vi "Last_check.vi"(3 "error in":errorcluster, 4 "Step Number in":i32, 5 "Data in":T1) -> (0 "error out":errorcluster, 1 "Step Number out":i32, 2 "Data out":T1)   [LabVIEW 2017, in "Steps.lvlib"]
uses:
  Steps.lvlib
  Type_Defs/Data.ctl
  Type_Defs/Diagnostics.ctl
  Type_Defs/Systems.ctl
panel:
  in  "Step Back":bool
  in  "Continue":bool
  out "All Systems Ready?":bool=TRUE
  # "Options"
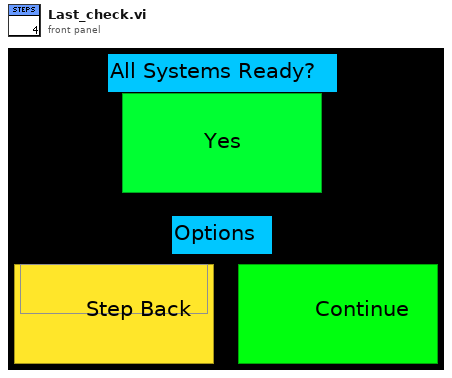
[diagram p1: front panel]
types:
  T1 = typedef "Data.ctl" = cluster{"User Name":string, "Experiment Number":i32, "Start Time":timestamp, "Data":dbl[], "Step Number":i32, "Step Instructions":string, "Diagnostics":T2, "Experiment Purpose":string, "Experiment State":enum16{"Off", "Setting Up", "Ready", "In Progress", "Shutting Down"}, "Systems":T3, "Vacuum Pressure":dbl, "Fieldpoints":cluster{"System Boolean Fieldpoints":cluster{"Compressed Air":refnum<k21>, "T-20kV Power Switch":refnum<k21>, "T-Rectifier":refnum<k21>, "Engage Interlock":refnum<k21>, "Ventilator":refnum<k21>, "Magnetron":refnum<k21>, "H-20kV Power Switch":refnum<k21>, "H-Rectifier":refnum<k21>, "Main Water Pump":refnum<k21>, "WEGA Water Pump":refnum<k21>, "Gas Inlet Valves":refnum<k21>}, "Step Fieldpoints":cluster{"Exhaust Ventillator":refnum<k21>, "Compressed Air":refnum<k21>, "Water Pressure":refnum<k21>, "Interlock":refnum<k21>, "Toroidal Power Supply 1":refnum<k21>, "Toroidal Power Supply 2":refnum<k21>, "Toroidal Rectifier":refnum<k21>, "Helical Power Supply":refnum<k21>, "Helical Rectifier":refnum<k21>, "6kW Magnetron Standby":refnum<k21>, "20kW Magnetron Standby":refnum<k21>}}, "Pressure History":cluster{"Seconds into Experiment":i32[], "Pressure Data":dbl[]}, "Time Computer Control":dbl[], "Toroidal Voltage Computer Control":dbl[], "Helical Voltage Computer Control":dbl[], "Toroidal Current":dbl[], "Toroidal Voltage":dbl[], "Toroidal Current Set Point":dbl[], "Helical Current Set Point":dbl[], "Helical Voltage":dbl[], "Helical Current":dbl[]}
  T2 = typedef "Diagnostics.ctl" = cluster{"Langmuir Probe":bool, "Rogowski 1":bool, "Rogowski 2":bool, "Rogowski 3":bool, "B-dot 1":bool, "B-dot 2":bool}
  T3 = typedef "Systems.ctl" = cluster{"Compressed Air":bool, "T-20kV Power Switch":bool, "T-Rectifier":bool, "Engage Interlock":bool, "Ventilator":bool, "Magnetron":bool, "H-20kV Power Switch":bool, "H-Rectifier":bool, "Main Water Pump":bool, "WEGA Water Pump":bool, "Gas Inlet Valves":bool}
  T4 = enum16{"Off", "Setting Up", "Ready", "In Progress", "Shutting Down"}
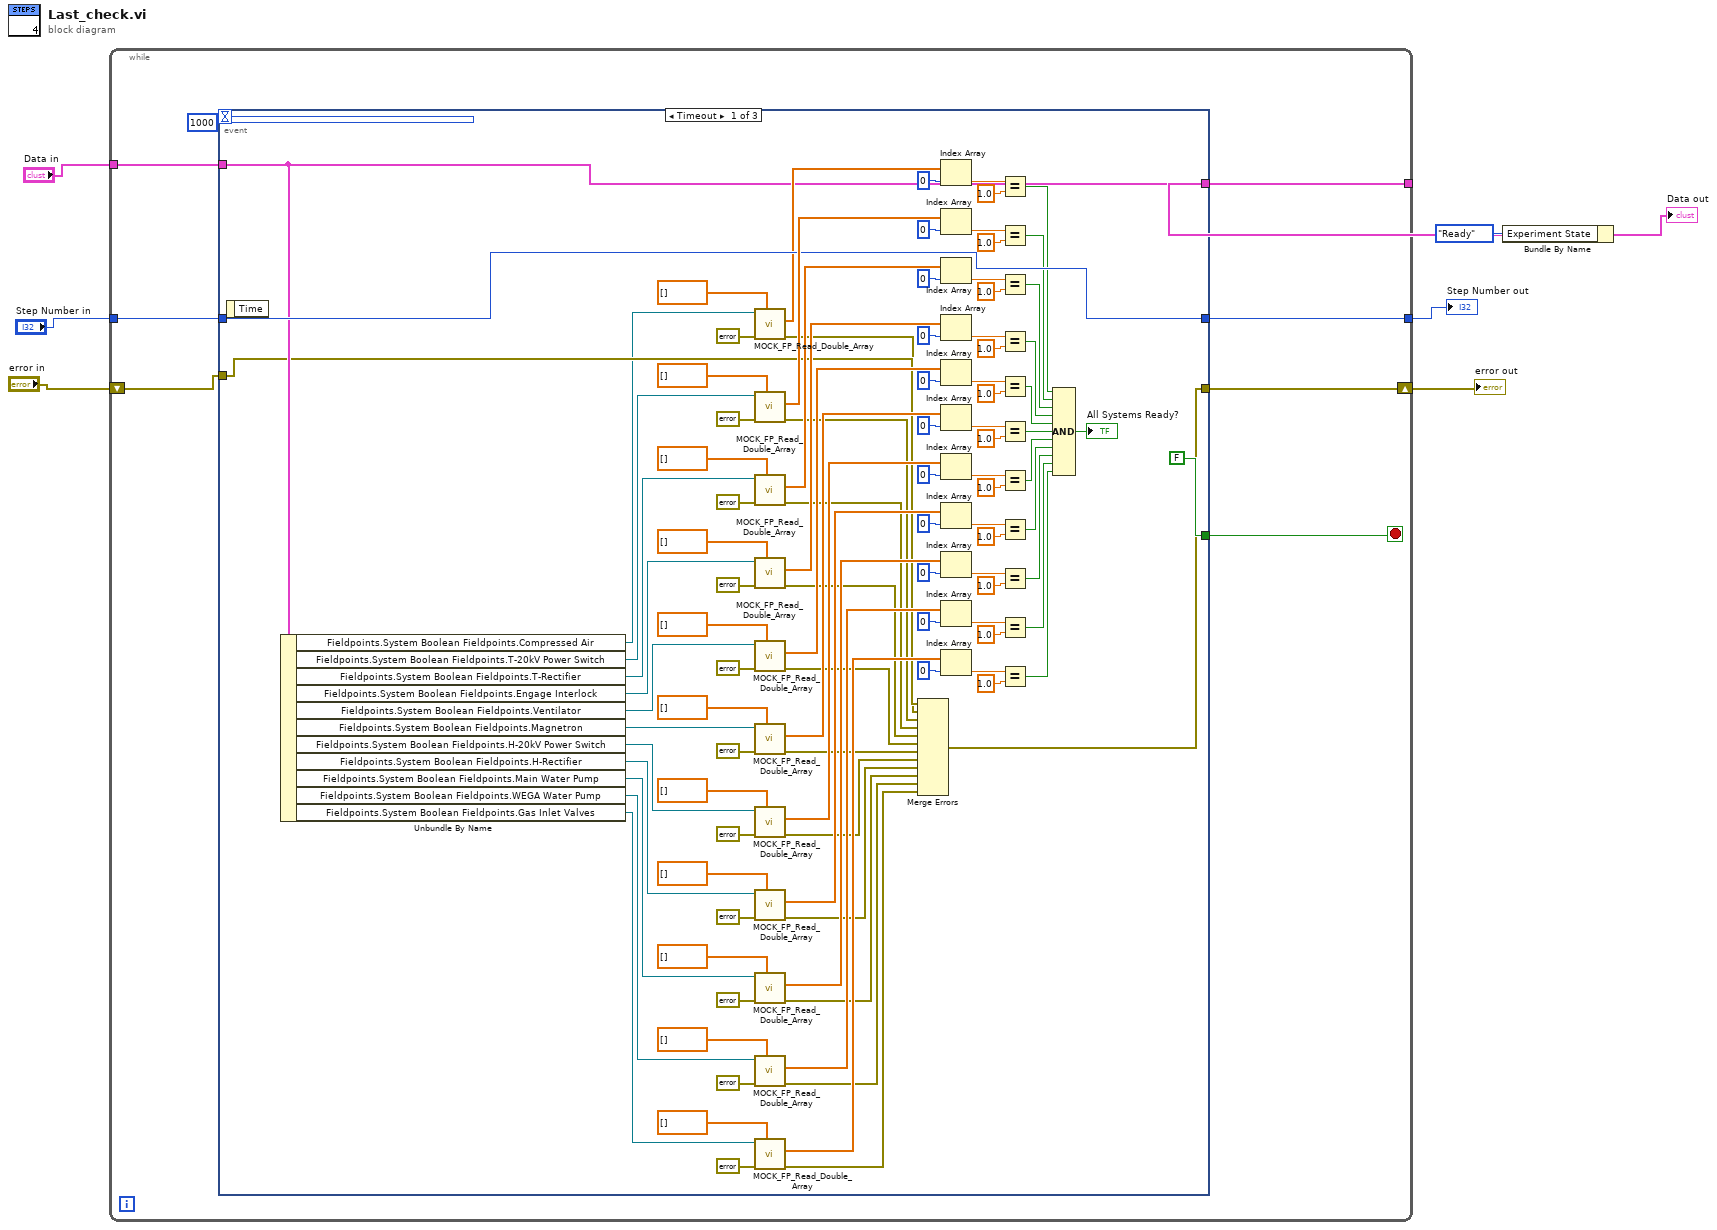
[diagram p0: block diagram]
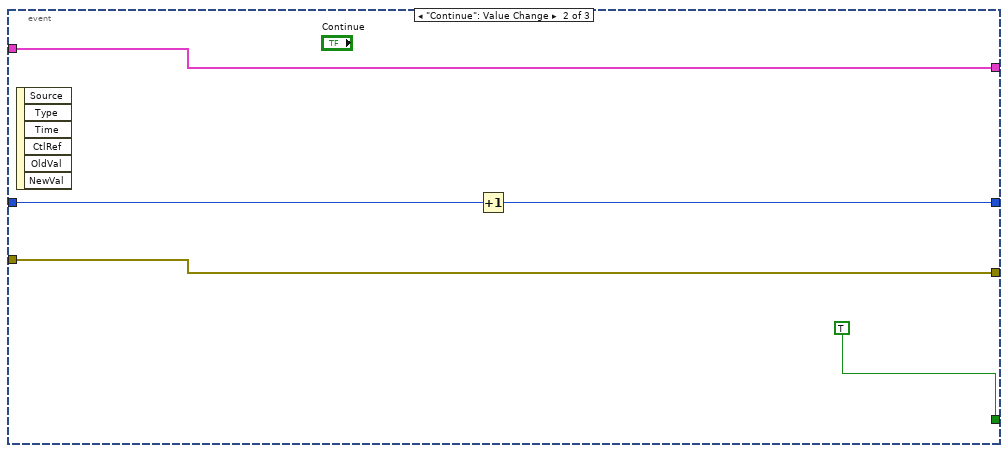
[diagram p2: hidden frame]
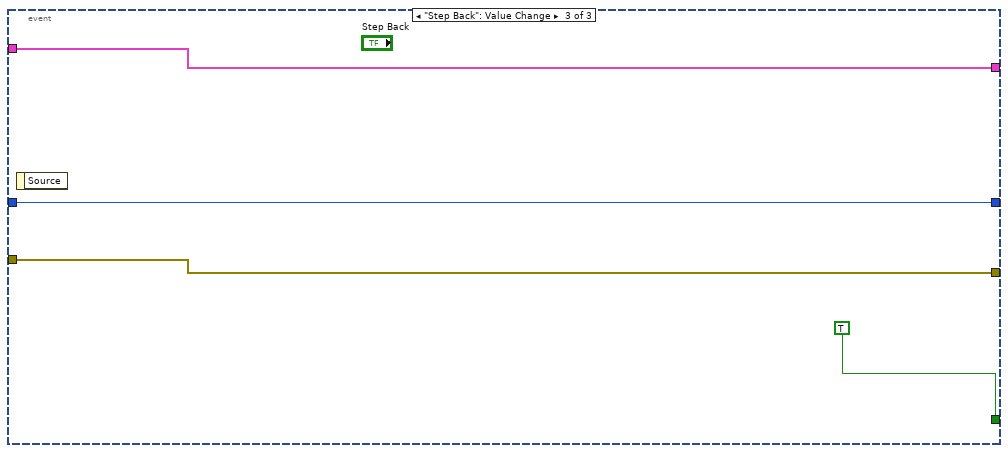
[diagram p3: hidden frame]
diagram:
  n1 = while {
    tunnel: [w12] -> w3
    tunnel: "Data in" -> [w11]
    tunnel: [w10] -> w6
    tunnel: "Step Number in" -> [w9]
    shift-right: [w14] -> w7
    shift-left: "error in" -> [w15]
    stop <- w13 stop-if-true
    n2 = event shown="[0] Timeout" {
      selector: _ -> [_ _ _]
      dyn-events: _ -> [_ _ _]
      timeout: 1000 -> [_ _ _]
      tunnel: w15 -> [w63 w125 w129]
      tunnel: [w62 w125 w129] -> w14
      tunnel: [FALSE TRUE TRUE] -> w13
      tunnel: [w64 w126 w130] -> w12
      tunnel: w11 -> [w64 w126 w130]
      tunnel: [w117 w123 w128] -> w10
      tunnel: w9 -> [w117 w124 w128]
      event Timeout {
        n3 = event-data() -> ()  [unwired: 1 in, 1 out]
        n4 = Unbundle By Name(w64) -> ("Fieldpoints.System Boolean Fieldpoints.Compressed Air"=w61:refnum<k21>, "Fieldpoints.System Boolean Fieldpoints.T-20kV Power Switch"=w60:refnum<k21>, "Fieldpoints.System Boolean Fieldpoints.T-Rectifier"=w59:refnum<k21>, "Fieldpoints.System Boolean Fieldpoints.Engage Interlock"=w58:refnum<k21>, "Fieldpoints.System Boolean Fieldpoints.Ventilator"=w57:refnum<k21>, "Fieldpoints.System Boolean Fieldpoints.Magnetron"=w56:refnum<k21>, "Fieldpoints.System Boolean Fieldpoints.H-20kV Power Switch"=w55:refnum<k21>, "Fieldpoints.System Boolean Fieldpoints.H-Rectifier"=w54:refnum<k21>, "Fieldpoints.System Boolean Fieldpoints.Main Water Pump"=w53:refnum<k21>, "Fieldpoints.System Boolean Fieldpoints.WEGA Water Pump"=w52:refnum<k21>, "Fieldpoints.System Boolean Fieldpoints.Gas Inlet Valves"=w51:refnum<k21>)
        n5 = call "MOCK_FP_Read_Double_Array.vi"("Type"=dbl[] [], "error in"=errorcluster {"status"=FALSE, "code"=0, "source"=""}, "FieldPoint IO Point In"=w61) -> ("error out"=w49:errorcluster, "Array"=w100:dbl[])  [unwired: 5 in, 2 out]
        n6 = call "MOCK_FP_Read_Double_Array.vi"("Type"=dbl[] [], "error in"=errorcluster {"status"=FALSE, "code"=0, "source"=""}, "FieldPoint IO Point In"=w60) -> ("error out"=w48:errorcluster, "Array"=w121:dbl[])  [unwired: 5 in, 2 out]
        n7 = call "MOCK_FP_Read_Double_Array.vi"("Type"=dbl[] [], "error in"=errorcluster {"status"=FALSE, "code"=0, "source"=""}, "FieldPoint IO Point In"=w59) -> ("error out"=w47:errorcluster, "Array"=w110:dbl[])  [unwired: 5 in, 2 out]
        n8 = call "MOCK_FP_Read_Double_Array.vi"("Type"=dbl[] [], "error in"=errorcluster {"status"=FALSE, "code"=0, "source"=""}, "FieldPoint IO Point In"=w58) -> ("error out"=w46:errorcluster, "Array"=w109:dbl[])  [unwired: 5 in, 2 out]
        n9 = call "MOCK_FP_Read_Double_Array.vi"("Type"=dbl[] [], "error in"=errorcluster {"status"=FALSE, "code"=0, "source"=""}, "FieldPoint IO Point In"=w57) -> ("error out"=w45:errorcluster, "Array"=w99:dbl[])  [unwired: 5 in, 2 out]
        n10 = call "MOCK_FP_Read_Double_Array.vi"("Type"=dbl[] [], "error in"=errorcluster {"status"=FALSE, "code"=0, "source"=""}, "FieldPoint IO Point In"=w56) -> ("error out"=w44:errorcluster, "Array"=w90:dbl[])  [unwired: 5 in, 2 out]
        n11 = call "MOCK_FP_Read_Double_Array.vi"("Type"=dbl[] [], "error in"=errorcluster {"status"=FALSE, "code"=0, "source"=""}, "FieldPoint IO Point In"=w55) -> ("error out"=w43:errorcluster, "Array"=w89:dbl[])  [unwired: 5 in, 2 out]
        n12 = call "MOCK_FP_Read_Double_Array.vi"("Type"=dbl[] [], "error in"=errorcluster {"status"=FALSE, "code"=0, "source"=""}, "FieldPoint IO Point In"=w54) -> ("error out"=w42:errorcluster, "Array"=w80:dbl[])  [unwired: 5 in, 2 out]
        n13 = call "MOCK_FP_Read_Double_Array.vi"("Type"=dbl[] [], "error in"=errorcluster {"status"=FALSE, "code"=0, "source"=""}, "FieldPoint IO Point In"=w53) -> ("error out"=w41:errorcluster, "Array"=w79:dbl[])  [unwired: 5 in, 2 out]
        n14 = call "MOCK_FP_Read_Double_Array.vi"("Type"=dbl[] [], "error in"=errorcluster {"status"=FALSE, "code"=0, "source"=""}, "FieldPoint IO Point In"=w52) -> ("error out"=w40:errorcluster, "Array"=w70:dbl[])  [unwired: 5 in, 2 out]
        n15 = call "MOCK_FP_Read_Double_Array.vi"("Type"=dbl[] [], "error in"=errorcluster {"status"=FALSE, "code"=0, "source"=""}, "FieldPoint IO Point In"=w51) -> ("error out"=w39:errorcluster, "Array"=w69:dbl[])  [unwired: 5 in, 2 out]
        n16 = Merge Errors(w63, w49, w48, w47, w46, w45, w44, w43, w42, w41, w40, w39) -> (w62:errorcluster)
        n17 = Index Array(array=w100, index=0) -> (element=w102:dbl)
        n18 = Index Array(array=w121, index=0) -> (element=w119:dbl)
        n19 = Index Array(array=w110, index=0) -> (element=w112:dbl)
        n20 = Index Array(array=w109, index=0) -> (element=w107:dbl)
        n21 = Index Array(array=w99, index=0) -> (element=w97:dbl)
        n22 = Index Array(array=w90, index=0) -> (element=w92:dbl)
        n23 = Index Array(array=w89, index=0) -> (element=w87:dbl)
        n24 = Index Array(array=w80, index=0) -> (element=w82:dbl)
        n25 = Index Array(array=w79, index=0) -> (element=w77:dbl)
        n26 = Index Array(array=w70, index=0) -> (element=w72:dbl)
        n27 = Index Array(array=w69, index=0) -> (element=w67:dbl)
        n28 = Equal?(x=w102, y=1.0) -> (x = y?=w28:bool)
        n29 = Equal?(x=w119, y=1.0) -> (x = y?=w27:bool)
        n30 = Equal?(x=w112, y=1.0) -> (x = y?=w26:bool)
        n31 = Equal?(x=w107, y=1.0) -> (x = y?=w25:bool)
        n32 = Equal?(x=w97, y=1.0) -> (x = y?=w24:bool)
        n33 = Equal?(x=w92, y=1.0) -> (x = y?=w23:bool)
        n34 = Equal?(x=w87, y=1.0) -> (x = y?=w22:bool)
        n35 = Equal?(x=w82, y=1.0) -> (x = y?=w21:bool)
        n36 = Equal?(x=w77, y=1.0) -> (x = y?=w20:bool)
        n37 = Equal?(x=w72, y=1.0) -> (x = y?=w19:bool)
        n38 = Equal?(x=w67, y=1.0) -> (x = y?=w18:bool)
        n39 = Compound Arithmetic op=AND(w28, w27, w26, w25, w24, w23, w22, w21, w20, w19, w18) -> (→"All Systems Ready?":bool)
      }
      event "Continue": Value Change {
        n40 = event-data() -> ()  [unwired: 1 in, 6 out]
        n41 = Increment(x=w124) -> (x+1=w123:i32)
      }
      event "Step Back": Value Change {
        n42 = event-data() -> ()  [unwired: 1 in, 1 out]
      }
    }
  }
  "error out" <- w7
  "Step Number out" <- w6
  n43 = Bundle By Name(cluster=w3, "Experiment State"=T4."Ready") -> (→"Data out":T1)
